vi "创建宏命令.vi"(8 "error in (no error)":errorcluster caption="错误输入（无错误）", 10 "宏命令":refnum<class "命令类.lvclass">[](array[class]), 11 "控制盒（宏命令） 输入":refnum<class "控制盒（宏命令）.lvclass"> caption="DNL_LabVIEW Object in") -> (0 "error out":errorcluster caption="错误输出", 3 "控制盒（宏命令） 输出":refnum<class "控制盒（宏命令）.lvclass"> caption="DNL_LabVIEW Object out")   [LabVIEW 2011, in "控制盒（宏命令）.lvclass"]
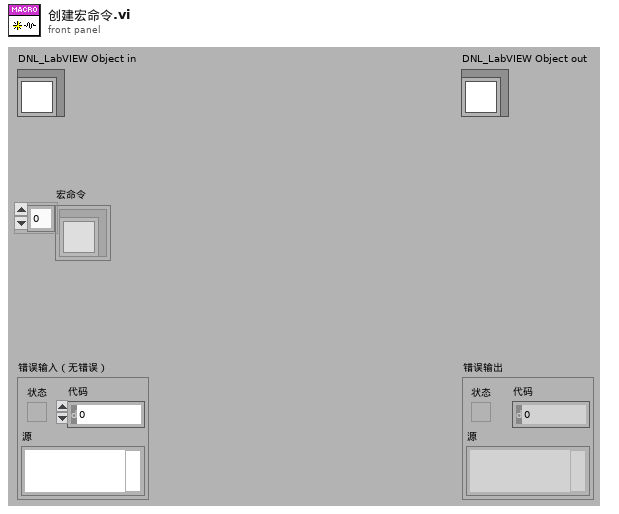
[diagram p1: front panel]
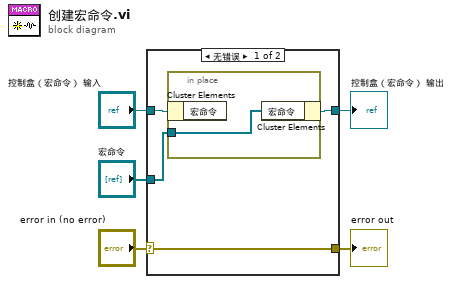
[diagram p0: block diagram]
diagram:
  n1 = case shown="无错误" "error in (no error)" {
    selector: "error in (no error)" -> [w9 w12]
    tunnel: [w9 w12] -> w4
    tunnel: [w6 w11] -> w2
    tunnel: "控制盒（宏命令） 输入" -> [w8 w11]
    tunnel: "宏命令" -> [w7 _]
    frame No Error {
      n2 = in-place {
        in-place-border: w7 -> [w10]
        n3 = in-place-cluster #1(w8) -> ()  [unwired: 1 out]
        n4 = in-place-cluster #1("宏命令"=w10) -> (w6:refnum<class "控制盒（宏命令）.lvclass">)
      }
    }
    frame Error {
    }
  }
  "error out" <- w4
  "控制盒（宏命令） 输出" <- w2
